vi "Search File Name.vi"(10 "File Path In":path) -> (1 "File name found?":bool, 2 "File Path Out":path)   [LabVIEW 2018, in "File IO.lvlib"]
doc: "This VI searches for the file name in the file path and outputs a boolean for whether or not file name was found."
uses:
  File IO.lvlib
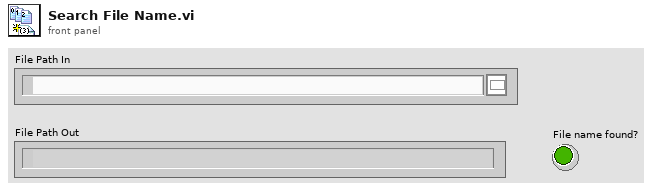
[diagram p1: front panel]
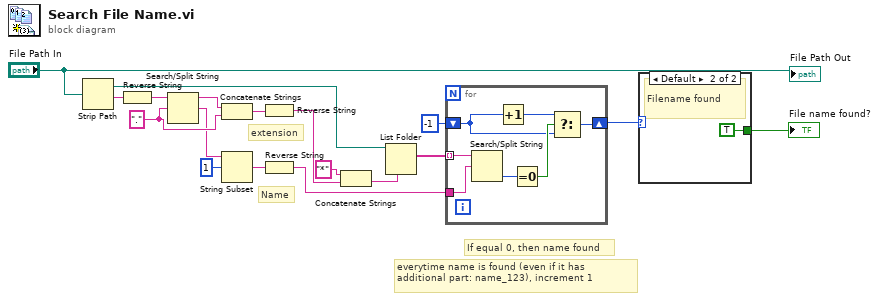
[diagram p0: block diagram]
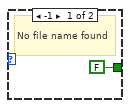
[diagram p2: hidden frame]
diagram:
  w14 = "." ("search string/char (-)")
  # "extension"
  # "Name"
  # "everytime name is found (even if it has additional part: name_123), increment 1"
  # "If equal 0, then name found"
  n1 = Strip Path(path="File Path In") -> (stripped path=w4:path, name=w8:string)
  n2 = Reverse String(1:w8) -> (0:w9:string)
  n3 = Search/Split String(string=w9, search string/char (-)=w14) -> (substring before match=w13:string, match + rest of string=w10:string)  [unwired: 1 in, 1 out]
  n4 = Concatenate Strings(w13, w14) -> (w15:string)
  n5 = String Subset(string=w10, offset (0)=1) -> (substring=w12:string)  [unwired: 1 in]
  n6 = Reverse String(1:w15) -> (0:w5:string)
  n7 = Reverse String(1:w12) -> (0:w6:string)
  n8 = Concatenate Strings("*" ("string"), w5) -> (w7:string)
  n9 = List Folder(path=w4, pattern=w7) -> (filenames=w18:string[])  [unwired: 2 in, 3 out]
  n10 = for {
    tunnel: w18 -> [w25] mode=indexing
    shift-right: [w23] -> w1
    shift-left: -1 -> [w21]
    tunnel: w6 -> [w19]
    n11 = Search/Split String(string=w25, search string/char (-)=w19) -> (offset of match=w24:i32)  [unwired: 1 in, 2 out]
    n12 = Increment(x=w21) -> (x+1=w20:i32)
    n13 = Equal To 0?(x=w24) -> (x = 0?=w22:bool)
    n14 = Select(t=w20, s=w22, f=w21) -> (s? t:f=w23:i32)
  }
  n15 = case shown="Default" w1 {
    tunnel: [FALSE ("Filename found?") TRUE ("Filename found?")] -> w3
    frame -1 {
      # "No file name found"
    }
    frame Default {
      # "Filename found"
    }
  }
  "File name found?" <- w3
  "File Path Out" <- "File Path In"
